vi "DP-Append Raw Data File.vi"(0 "raw file":path, 5 "freq":dbl[](array[numeric]), 7 "ntime":i32, 9 "nfreq":i32, 11 "error in (no error)":errorcluster) -> (4 "Byte Stream File out":refnum<file>, 15 "error out":errorcluster)   [LabVIEW 2020]
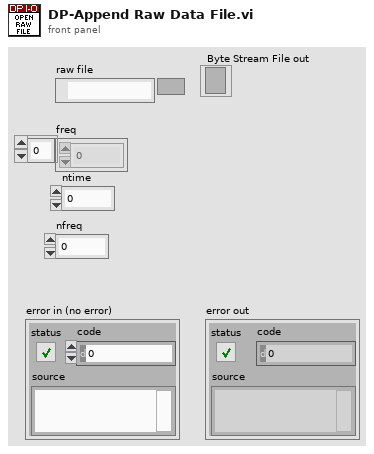
[diagram p1: front panel]
types:
  T1 = enum16{"open", "replace", "create", "open or create", "replace or create", "replace or create with confirmation"}
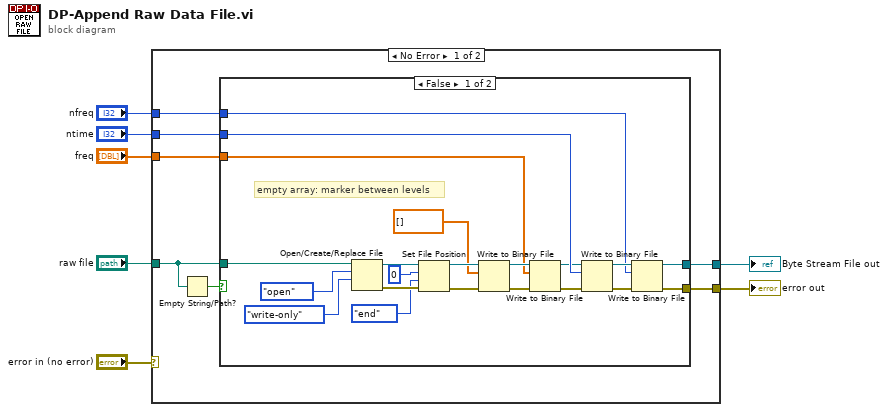
[diagram p0: block diagram]
diagram:
  n1 = case shown="No Error" "error in (no error)" {
    selector: "error in (no error)" -> [_ w36]
    tunnel: "raw file" -> [w9 _]
    tunnel: "freq" -> [w14 _]
    tunnel: "ntime" -> [w13 _]
    tunnel: "nfreq" -> [w12 _]
    tunnel: [w11 w36] -> w3
    tunnel: [w10 _] -> w2
    frame No Error {
      n2 = Empty String/Path?(string/path=w9) -> (empty?=w8:bool)
      n3 = case shown="False" w8 {
        tunnel: w9 -> [w35 _]
        tunnel: w14 -> [w23 _]
        tunnel: w13 -> [w21 _]
        tunnel: w12 -> [w17 _]
        tunnel: [w16 _] -> w11
        tunnel: [w15 _] -> w10
        frame False {
          # "empty array: marker between levels"
          n4 = Open/Create/Replace File(file path (use dialog)=w35, operation (0:open)=T1."open", access (0:read/write)=enum16{"read/write", "read-only", "write-only"}."write-only") -> (refnum out=w32:refnum<file>, error out=w31:errorcluster)  [unwired: 3 in, 1 out]
          n5 = Set File Position(offset (in bytes) (0)=i64 0, refnum=w32, from (0:start)=enum16{"start", "end", "current"}."end", error in=w31) -> (refnum out=w27:refnum<file>, error out=w28:errorcluster)
          n6 = Write to Binary File(file (use dialog)=w27, data=dbl[] [], error in=w28) -> (refnum out=w25:refnum<file>, error out=w24:errorcluster)  [unwired: 3 in, 1 out]
          n7 = Write to Binary File(file (use dialog)=w25, data=w23, error in=w24) -> (refnum out=w19:refnum<file>, error out=w22:errorcluster)  [unwired: 3 in, 1 out]
          n8 = Write to Binary File(file (use dialog)=w19, data=w21, error in=w22) -> (refnum out=w18:refnum<file>, error out=w20:errorcluster)  [unwired: 3 in, 1 out]
          n9 = Write to Binary File(file (use dialog)=w18, data=w17, error in=w20) -> (refnum out=w15:refnum<file>, error out=w16:errorcluster)  [unwired: 3 in, 1 out]
        }
        frame True {
        }
      }
    }
    frame Error {
    }
  }
  "error out" <- w3
  "Byte Stream File out" <- w2
